vi "niRFUtil WFM Decimate Waveform (real wfm).vi"(0 "Waveform In":T1 {"y" min=0 max=127 format="%.2f"; "dx" format="%^.2e"; "x0" format="%^.2e"}, 5 "Rate (1)":i32=1, 7 "Offset (0)":i32, 13 "Average? (F)":bool) -> (4 "Waveform Out":T1 {"y" min=0 max=127 format="%.2f"; "dx" format="%^.2e"; "x0" format="%^.2e"})   [LabVIEW 2015, in "niRFUtil.lvlib"]
doc: "(c) Copyright 2006, National Instruments, Inc. This VI may not be duplicated, sold, or distributed without written consent from National Instruments."
uses:
  niRFUtil.lvlib
  Includes/niRFUtil INC Real Waveform.ctl
  Includes/niRFUtil INC Real Array.ctl
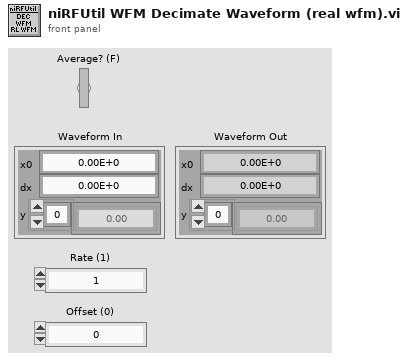
[diagram p1: front panel]
types:
  T1 = typedef "niRFUtil.lvlib/niRFUtil INC Real Waveform.ctl" = cluster{"x0":dbl, "dx":dbl, "y":T2}
  T2 = typedef "niRFUtil.lvlib/niRFUtil INC Real Array.ctl" = sgl[]
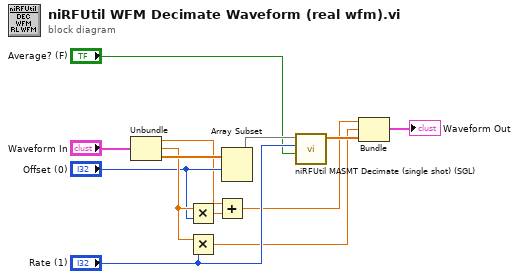
[diagram p0: block diagram]
diagram:
  n1 = Unbundle("Waveform In") -> ("x0"=w4:dbl, "dx"=w7:dbl, "y"=w11:T2)
  n2 = Multiply(x=w7, y="Offset (0)") -> (x*y=w5:dbl)
  n3 = Multiply(x=w7, y="Rate (1)") -> (x*y=w8:dbl)
  n4 = Add(x=w4, y=w5) -> (x+y=w3:dbl)
  n5 = Array Subset(array=w11, index="Offset (0)") -> (w12:T2)  [unwired: 1 in]
  n6 = call "niRFUtil MASMT Decimate (single shot) (SGL).vi"("averaging"="Average? (F)", "decimating factor"="Rate (1)", "X"=w12) -> ("Decimated X"=w10:sgl[])  [unwired: 7 in, 1 out]
  n7 = Bundle(w3, w8, "Decimated X"=w10) -> (→"Waveform Out":cluster{dbl, dbl, "Decimated X":sgl[]})  [unwired: 1 out]
